vi "WavetoXYData.vi"   [LabVIEW 2014]
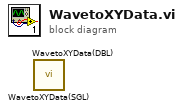
[diagram p0: block diagram]
diagram:
  n1 = call "WavetoXYData(SGL).vi"() -> ()  [unwired: 10 in, 2 out]
  n2 = call "WavetoXYData(DBL).vi"() -> ()  [unwired: 10 in, 2 out]
